vi "Cable Length Plot.vi"(9 "Motor Config X":dbl[](array[numeric]), 10 "Motor Config Y":dbl[](array[numeric]), 11 "Cable Length":dbl[](array[numeric])) -> (1 "Circle 3":cluster{dbl[], dbl[]}, 2 "Circle 2":cluster{dbl[], dbl[]}, 3 "Circle 1":cluster{dbl[], dbl[]})   [LabVIEW 2021]
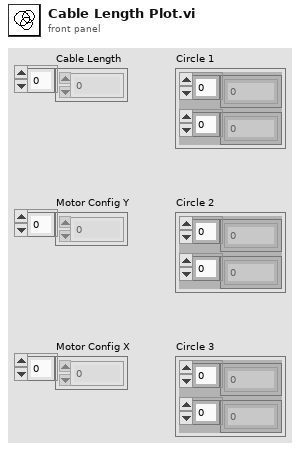
[diagram p1: front panel]
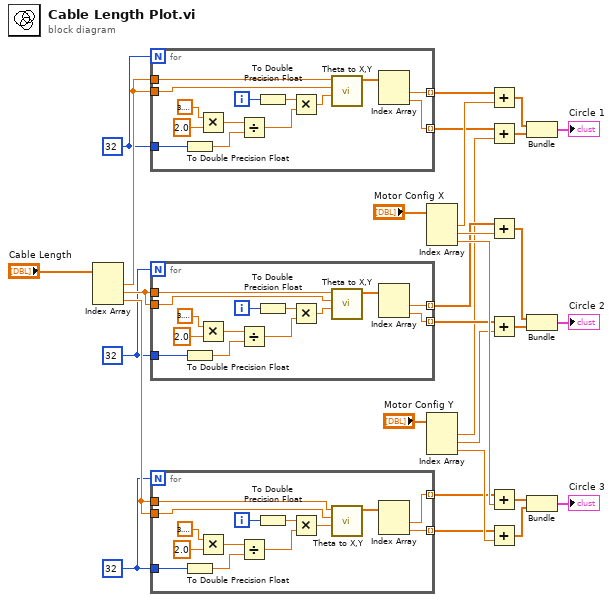
[diagram p0: block diagram]
diagram:
  w15 = 32 ("Drawing Samples")
  w12 = 32 ("Drawing Samples")
  w1 = 32 ("Drawing Samples")
  n1 = Index Array(array="Cable Length") -> (element #1=w4:dbl, element #2=w18:dbl, element #3=w19:dbl)  [unwired: 3 in]
  n2 = for {
    N: w1 -> [_]
    tunnel: [w35] -> w2 mode=indexing
    tunnel: [w34] -> w3 mode=indexing
    tunnel: w1 -> [w42]
    tunnel: w4 -> [w38]
    tunnel: w4 -> [w37]
    i -> [w43]
    n3 = To Double Precision Float(number=w42) -> (double precision float=w40:dbl)
    n4 = Multiply(x=3.141592653589793, y=2.0 ("x")) -> (x*y=w31:dbl)
    n5 = Divide(x=w31, y=w40) -> (x/y=w44:dbl)
    n6 = To Double Precision Float(number=w43) -> (double precision float=w41:dbl)
    n7 = Multiply(x=w41, y=w44) -> (x*y=w39:dbl)
    n8 = call "Theta to X,Y.vi"("theta"=w39, "b"=w37, "a"=w38) -> ("X,Y"=w36:dbl[])  [unwired: 8 in]
    n9 = Index Array(array=w36) -> (element #1=w35:dbl, element #2=w34:dbl)  [unwired: 2 in]
  }
  n10 = for {
    N: w12 -> [_]
    tunnel: [w49] -> w13 mode=indexing
    tunnel: [w48] -> w14 mode=indexing
    tunnel: w12 -> [w56]
    tunnel: w18 -> [w52]
    tunnel: w18 -> [w51]
    i -> [w57]
    n11 = To Double Precision Float(number=w56) -> (double precision float=w54:dbl)
    n12 = Multiply(x=3.141592653589793, y=2.0 ("x")) -> (x*y=w45:dbl)
    n13 = Divide(x=w45, y=w54) -> (x/y=w58:dbl)
    n14 = To Double Precision Float(number=w57) -> (double precision float=w55:dbl)
    n15 = Multiply(x=w55, y=w58) -> (x*y=w53:dbl)
    n16 = call "Theta to X,Y.vi"("theta"=w53, "b"=w51, "a"=w52) -> ("X,Y"=w50:dbl[])  [unwired: 8 in]
    n17 = Index Array(array=w50) -> (element #1=w49:dbl, element #2=w48:dbl)  [unwired: 2 in]
  }
  n18 = for {
    N: w15 -> [_]
    tunnel: [w63] -> w16 mode=indexing
    tunnel: [w62] -> w17 mode=indexing
    tunnel: w15 -> [w70]
    tunnel: w19 -> [w66]
    tunnel: w19 -> [w65]
    i -> [w71]
    n19 = To Double Precision Float(number=w70) -> (double precision float=w68:dbl)
    n20 = Multiply(x=3.141592653589793, y=2.0 ("x")) -> (x*y=w59:dbl)
    n21 = Divide(x=w59, y=w68) -> (x/y=w72:dbl)
    n22 = To Double Precision Float(number=w71) -> (double precision float=w69:dbl)
    n23 = Multiply(x=w69, y=w72) -> (x*y=w67:dbl)
    n24 = call "Theta to X,Y.vi"("theta"=w67, "b"=w65, "a"=w66) -> ("X,Y"=w64:dbl[])  [unwired: 8 in]
    n25 = Index Array(array=w64) -> (element #1=w63:dbl, element #2=w62:dbl)  [unwired: 2 in]
  }
  n26 = Index Array(array="Motor Config X") -> (element #1=w7:dbl, element #2=w20:dbl, element #3=w22:dbl)  [unwired: 3 in]
  n27 = Index Array(array="Motor Config Y") -> (element #1=w8:dbl, element #2=w21:dbl, element #3=w23:dbl)  [unwired: 3 in]
  n28 = Add(x=w2, y=w7) -> (x+y=w9:dbl[])
  n29 = Add(x=w3, y=w8) -> (x+y=w10:dbl[])
  n30 = Add(x=w13, y=w20) -> (x+y=w24:dbl[])
  n31 = Add(x=w14, y=w21) -> (x+y=w25:dbl[])
  n32 = Add(x=w16, y=w22) -> (x+y=w26:dbl[])
  n33 = Add(x=w17, y=w23) -> (x+y=w27:dbl[])
  n34 = Bundle(w9, w10) -> (→"Circle 1":cluster{dbl[], dbl[]})  [unwired: 1 in]
  n35 = Bundle(w24, w25) -> (→"Circle 2":cluster{dbl[], dbl[]})  [unwired: 1 in]
  n36 = Bundle(w26, w27) -> (→"Circle 3":cluster{dbl[], dbl[]})  [unwired: 1 in]
